vi "Pixel Intensity Search.vi"() -> ()   [LabVIEW 2016]
uses:
  <vilib>/userdefined/High Color/IMAQdx.ctl
  <vilib>/vision/driver/NI_Vision_Acquisition_Software.lvlib
  <vilib>/vision/NI_Vision_Development_Module.lvlib
panel:
  out "max value":dbl
  out "size(s) 3":i32
  out "subarray":dbl[](array[numeric])
  out "size(s) 2":i32
  out "Array":dbl[](array[numeric])
  out "Array 2":u8[][](array[numeric])
  out "size(s)":i32
  in  "Number":i32
  out "error out":errorcluster
  in  "error in":errorcluster
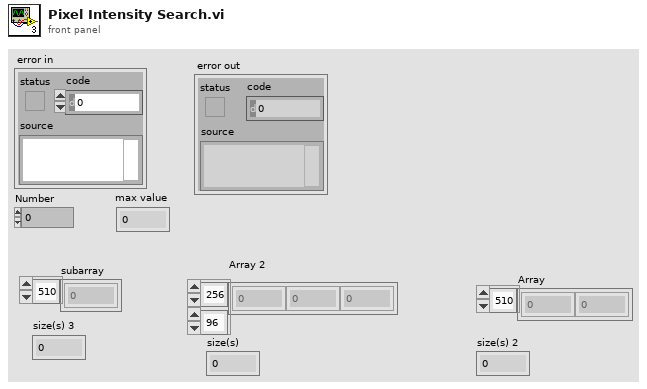
[diagram p1: front panel]
types:
  T1 = typedef "IMAQdx.ctl" = refnum<k21>
  T2 = typedef "IMAQ Image.ctl" = refnum<image>
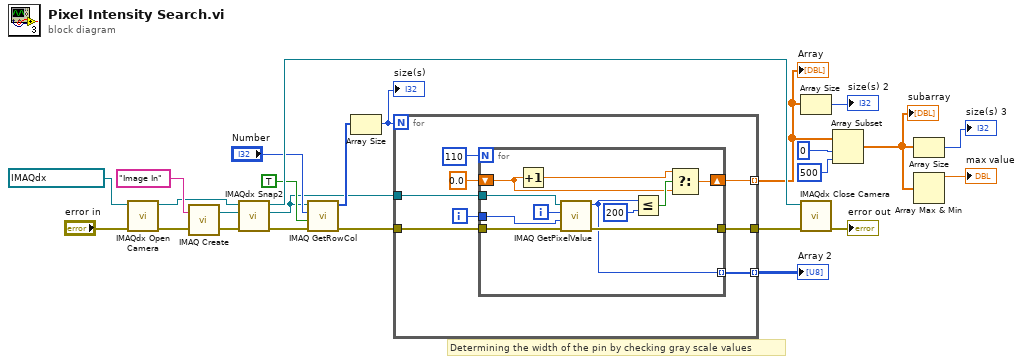
[diagram p0: block diagram]
diagram:
  # "Determining the width of the pin by checking gray scale values"
  n1 = call <vilib>:"IMAQdx Open Camera.vi"("error in"="error in", "Session In"=T1 "acA780-75gc") -> ("error out"=w23:errorcluster, "Session Out"=w19:T1)  [unwired: 8 in]
  n2 = call "IMAQ Create"("Image Name"="Image In", "error in (no error)"=w23) -> ("New Image"=w20:T2, "error out"=w21:errorcluster)  [unwired: 3 in]
  n3 = call <vilib>:"IMAQdx Snap2.vi"("error in"=w21, "Image In"=w20, "Session In"=w19) -> ("error out"=w14:errorcluster, "Image Out"=w11:T2, "Session Out"=w17:T1)  [unwired: 6 in]
  n4 = call "IMAQ GetRowCol"("Image"=w11, "Number"="Number", "Row / Column (Row)"=TRUE, "error in (no error)"=w14) -> ("Pixels (U8)"=w13:u8[], "error out"=w10:errorcluster)  [unwired: 2 in, 3 out]
  n5 = Array Size(array=w13) -> (size(s)=w12:i32)
  "size(s)" <- w12
  n6 = for {
    N: w12 -> [_]
    tunnel: w11 -> [w33]
    tunnel: w10 -> [w31]
    tunnel: [w30] -> w9
    tunnel: [w29] -> w7 mode=indexing
    tunnel: [w26] -> w4 mode=indexing
    i -> [w32]
    n7 = for {
      N: 110 -> [_]
      tunnel: w33 -> [w44]
      tunnel: w32 -> [w43]
      tunnel: w31 -> [w42]
      tunnel: [w41] -> w30
      tunnel: [w39] -> w29 mode=indexing
      shift-right: [w35] -> w26
      shift-left: 0.0 -> [w34]
      i -> [w40]
      n8 = Increment(x=w34) -> (x+1=w36:dbl)
      n9 = call "IMAQ GetPixelValue"("Image"=w44, "X Coordinate"=w40, "Y Coordinate"=w43, "error in (no error)"=w42) -> ("Pixel Value (U8)"=w39:u8, "error out"=w41:errorcluster)  [unwired: 2 in, 3 out]
      n10 = Less Or Equal?(x=w39, y=u8 200) -> (x <= y?=w38:bool)
      n11 = Select(t=w36, s=w38, f=w34) -> (s? t:f=w35:dbl)
    }
  }
  "Array 2" <- w7
  "Array" <- w4
  n12 = Array Size(array=w4) -> (size(s)=→"size(s) 2":i32)
  n13 = call <vilib>:"IMAQdx Close Camera.vi"("error in"=w9, "Session In"=w17) -> ("error out"=→"error out":errorcluster)  [unwired: 9 in]
  n14 = Array Subset(array=w4, index=0, length=500) -> (w2:dbl[])
  "subarray" <- w2
  n15 = Array Size(array=w2) -> (size(s)=→"size(s) 3":i32)
  n16 = Array Max & Min(array=w2) -> (max value=→"max value":dbl)  [unwired: 3 out]
